vi "Build Crosstalk Channel List.vi"(11 "Channel list":string[](array[string])) -> (3 "channel names":string[](array[string]))   [LabVIEW 2021, in "Crosstalk_Audio DAC.lvlib"]
uses:
  Crosstalk_Audio DAC.lvlib
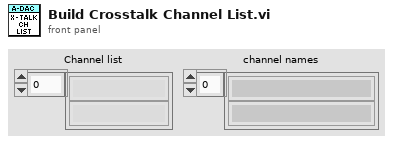
[diagram p1: front panel]
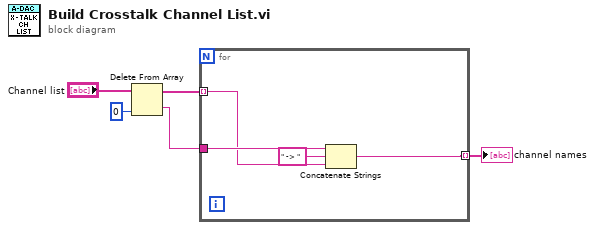
[diagram p0: block diagram]
diagram:
  n1 = Delete From Array(array="Channel list", index=0) -> (deleted portion=w2:string, array with subset deleted=w3:string[])  [unwired: 1 in]
  n2 = for {
    tunnel: w3 -> [w7] mode=indexing
    tunnel: w2 -> [w9]
    tunnel: [w6] -> w1 mode=indexing
    n3 = Concatenate Strings(w9, " -> " ("string"), w7) -> (w6:string)
  }
  "channel names" <- w1
